vi "Withdrawal.vi"(8 "error in (no error)":errorcluster, 11 "Amount":i32) -> (0 "error out":errorcluster, 3 "Successful?":bool)   [LabVIEW 2012]
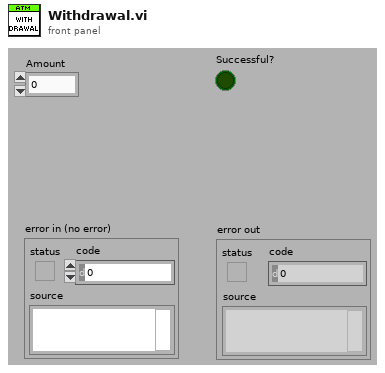
[diagram p1: front panel]
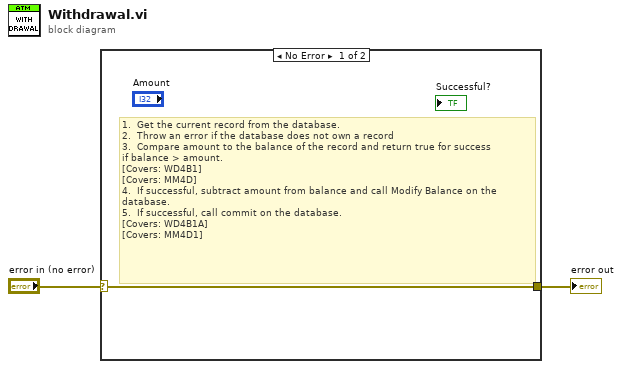
[diagram p0: block diagram]
diagram:
  n1 = case shown="No Error" "error in (no error)" {
    selector: "error in (no error)" -> [w3 w4]
    tunnel: [w3 w4] -> w1
    frame No Error {
      # "1.  Get the current record from the database.\n2.  Throw an error if the database does not own a record\n3.  Compare amount to the balance of the record and return true for success\nif balance > amount.\n[Covers: WD4B1]\n[Covers: MM4D]\n4.  If successful, subtract amount from balance and call Modify Balance on the\ndatabase.\n5.  If successful, call commit on the database.\n[Covers: WD4B1A]\n[Covers: MM4D1]"
    }
    frame Error {
    }
  }
  "error out" <- w1
